vi "Initialize.vi"(8 "error in":errorcluster, 10 "ID Query (True)":bool=TRUE, 11 "VISA resource name":refnum<visa-resource-name>) -> (0 "error out":errorcluster, 2 "Identity":T1, 3 "VISA resource name out":refnum<visa-resource-name>)   [LabVIEW 2020, in "HandsOnPi2040.lvlib"]
doc: "Establishes communication with the instrument and optionally performs an instrument identification query and/or an instrument reset. It also places the instrument in a default state needed for other instrument driver operations. Therefore, call this VI before calling other instrument driver VIs for this instrument. Generally, you need to call the <b>Initialize</b> VI only once at the beginning of an application."
uses:
  HandsOnPi2040.lvlib
  <vilib>/CTI/CTI Visa Drivers/CTI-Visa/Identity.ctl
  <vilib>/CTI/CTI Visa Drivers/CTI-Visa/Digital Direction.ctl
  <vilib>/CTI/CTI Visa Drivers/CTI-Visa/CTI-Visa.lvlib
panel:
  # "Input"
  # "Output"
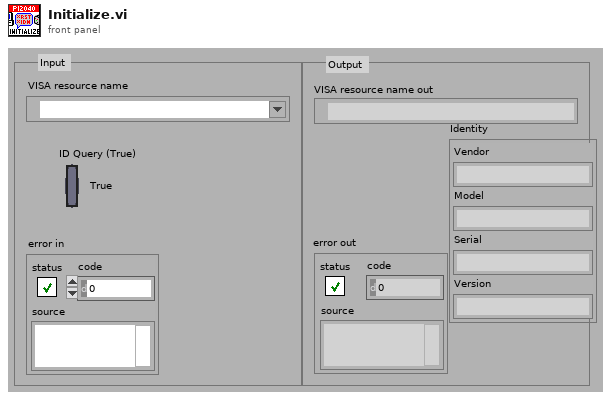
[diagram p1: front panel]
types:
  T1 = typedef "CTI-Visa.lvlib/Identity.ctl" = cluster{"Vendor":string, "Model":string, "Serial":string, "Version":string}
  T2 = typedef "CTI-Visa.lvlib/Digital Direction.ctl" = enum16{"In", "Out"}
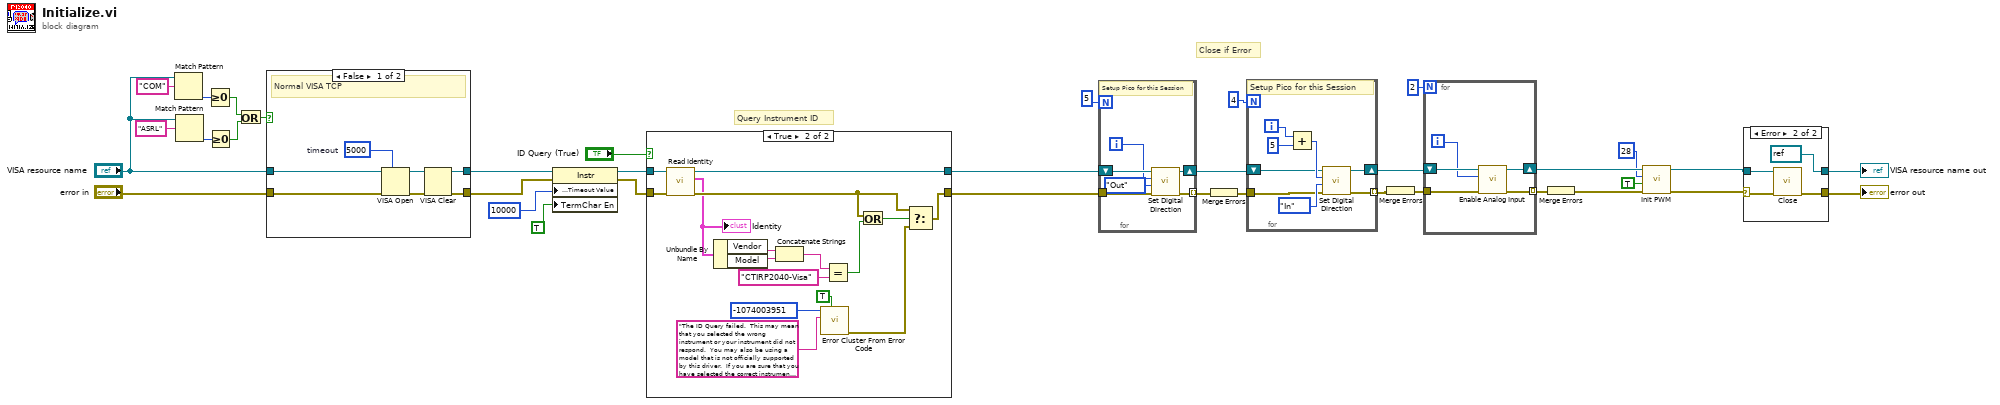
[diagram p0: block diagram]
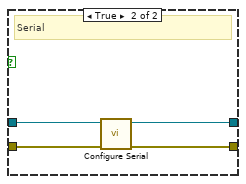
[diagram p2: hidden frame]
diagram:
  # "Close if Error"
  # "Query Instrument ID"
  n1 = Match Pattern(string="VISA resource name", regular expression="COM") -> (offset past match=w25:i32)  [unwired: 1 in, 3 out]
  n2 = Match Pattern(string="VISA resource name", regular expression="ASRL") -> (offset past match=w24:i32)  [unwired: 1 in, 3 out]
  n3 = Greater Or Equal To 0?(x=w25) -> (x >= 0?=w23:bool)
  n4 = Greater Or Equal To 0?(x=w24) -> (x >= 0?=w22:bool)
  n5 = Or(x=w23, y=w22) -> (x .or. y?=w21:bool)
  n6 = case shown="False" w21 {
    tunnel: "VISA resource name" -> [w43 w47]
    tunnel: "error in" -> [w42 w46]
    tunnel: [w38 w45] -> w19
    tunnel: [w37 w44] -> w20
    frame False {
      w41 = u32 5000  # timeout
      # "Normal VISA TCP"
      n7 = VISA Open(timeout (0)=w41, error in (no error)=w42, VISA resource name=w43) -> (VISA resource name=w40:refnum<visa-resource-name>, error out=w39:errorcluster)  [unwired: 2 in]
      n8 = VISA Clear(VISA resource name=w40, error in (no error)=w39) -> (VISA resource name out=w38:refnum<visa-resource-name>, error out=w37:errorcluster)
    }
    frame True {
      # "Serial"
      n9 = call <vilib>:"Configure Serial.vi"("error in (no error)"=w46, "VISA resource name in"=w47) -> ("error out"=w44:errorcluster, "VISA resource name"=w45:refnum<visa-resource-name>)  [unwired: 8 in]
    }
  }
  n10 = property class="Instr"(reference=w19, error in=w20, "General Settings:Timeout Value"=u32 10000, "TermChar En"=TRUE ("Message Based Settings:Termination Character Enable")) -> (reference out=w33:refnum<visa-resource-name>, error out=w32:errorcluster)
  n11 = case shown="True" "ID Query (True)" {
    tunnel: [w48 w65] -> w1
    tunnel: [w49 w59] -> w18
    tunnel: w33 -> [w49 w58]
    tunnel: w32 -> [w48 w57]
    frame False {
    }
    frame True {
      n12 = call <vilib>:"Read Identity.vi"("error in (no error)"=w57, "VISA resource name in"=w58) -> ("error out"=w56:errorcluster, "Identity"=w55:T1, "VISA resource name"=w59:refnum<visa-resource-name>)  [unwired: 7 in]
      "Identity" <- w55
      n13 = Unbundle By Name(w55) -> ("Vendor"=w53:string, "Model"=w54:string)
      n14 = Concatenate Strings(w53, w54) -> (w52:string)
      n15 = call <vilib>:"Error Cluster From Error Code.vi"("show call chain? (False)"=TRUE, "error message (\"\")"="The ID Query failed.  This may mean that you selected the wrong instrument or your instrument did not respond.  You may also be using a model that is not officially supported by this driver.  If you are sure that you have selected the correct instrument and it is responding, try disabling the ID Query." ("Source (VI Name)"), "error code (0)"=-1074003951 ("Code")) -> ("error out"=w64:errorcluster)  [unwired: 6 in]
      n16 = Equal?(x=w52, y="CTIRP2040-Visa") -> (x = y?=w50:bool)
      n17 = Or(x=w56, y=w50) -> (x .or. y?=w60:bool)
      n18 = Select(t=w56, s=w60, f=w64) -> (s? t:f=w65:errorcluster)
    }
  }
  n19 = for {
    N: 5 -> [_]
    shift-right: [w67] -> w10
    shift-left: w18 -> [w71]
    tunnel: w1 -> [w70]
    tunnel: [w66] -> w17 mode=indexing
    i -> [w68]
    # "Setup Pico for this Session"
    n20 = call <vilib>:"Set Digital Direction.vi"("error in (no error)"=w70, "Direction"=Digital_Direction."Out", "Channel"=w68, "VISA resource name in"=w71) -> ("error out"=w66:errorcluster, "VISA resource name"=w67:refnum<visa-resource-name>)  [unwired: 6 in]
  }
  n21 = Merge Errors(w17) -> (w11:errorcluster)
  n22 = for {
    N: 4 -> [_]
    shift-right: [w76] -> w9
    shift-left: w10 -> [w73]
    tunnel: [w75] -> w12 mode=indexing
    tunnel: w11 -> [w72]
    i -> [w74]
    # "Setup Pico for this Session"
    n23 = Add(x=w74, y=5) -> (x+y=w77:i32)
    n24 = call <vilib>:"Set Digital Direction.vi"("error in (no error)"=w72, "Direction"=Digital_Direction."In", "Channel"=w77, "VISA resource name in"=w73) -> ("error out"=w75:errorcluster, "VISA resource name"=w76:refnum<visa-resource-name>)  [unwired: 6 in]
  }
  n25 = Merge Errors(w12) -> (w13:errorcluster)
  n26 = for {
    N: 2 -> [_]
    shift-right: [w82] -> w7
    shift-left: w9 -> [w83]
    tunnel: w13 -> [w84]
    tunnel: [w81] -> w15 mode=indexing
    i -> [w80]
    n27 = call <vilib>:"Enable Analog Input.vi"("error in (no error)"=w84, "Channel"=w80, "VISA resource name in"=w83) -> ("error out"=w81:errorcluster, "VISA resource name"=w82:refnum<visa-resource-name>)  [unwired: 7 in]
  }
  n28 = Merge Errors(w15) -> (w6:errorcluster)
  n29 = call <vilib>:"Init PWM.vi"("error in (no error)"=w6, "Enable (F)"=TRUE, "Channel"=28, "VISA resource name in"=w7) -> ("error out"=w5:errorcluster, "VISA resource name"=w4:refnum<visa-resource-name>)  [unwired: 6 in]
  n30 = case shown="Error" w5 {
    selector: w5 -> [w85 w88]
    tunnel: w4 -> [w86 w89]
    tunnel: [w86 refnum<visa-resource-name> refnum ("VISA resource name out")] -> w31
    tunnel: [w85 w90] -> w30
    frame No Error {
    }
    frame Error {
      n31 = call "Close.vi"("error in"=w88, "VISA resource name"=w89) -> ("error out"=w90:errorcluster)  [unwired: 9 in]
    }
  }
  "VISA resource name out" <- w31
  "error out" <- w30
